vi "AutoSetLEDemands.vi"(8 "error in (no error)":errorcluster, 9 "SetExtendPositonDemand(in)":dbl, 10 "SetLIftPostionDemand(d)":dbl) -> (0 "error out":errorcluster)   [LabVIEW 2020]
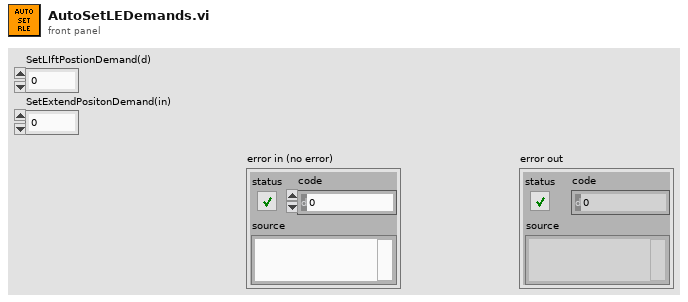
[diagram p1: front panel]
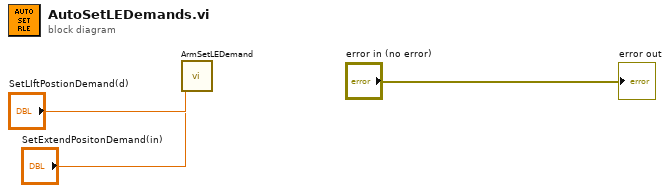
[diagram p0: block diagram]
diagram:
  n1 = call "ArmSetLEDemand.vi"("SetExtendPositonDemand(in)"="SetExtendPositonDemand(in)", "SetLIftPostionDemand(d)"="SetLIftPostionDemand(d)") -> ()  [unwired: 10 in]
  "error out" <- "error in (no error)"
